vi "Link.vi"(0 "Tosca in":refnum<class "Parameters.lvclass">, 11 "error in (no error)":errorcluster) -> (4 "Tosca out":refnum<class "Parameters.lvclass">, 15 "error out":errorcluster)   [LabVIEW 2020, in "Parameters.lvclass"]
uses:
  Parameters.lvclass
  Parameters.lvclass/Parameters.ctl
  State/State.lvclass
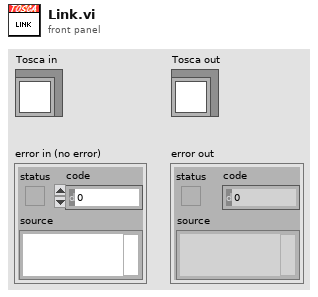
[diagram p1: front panel]
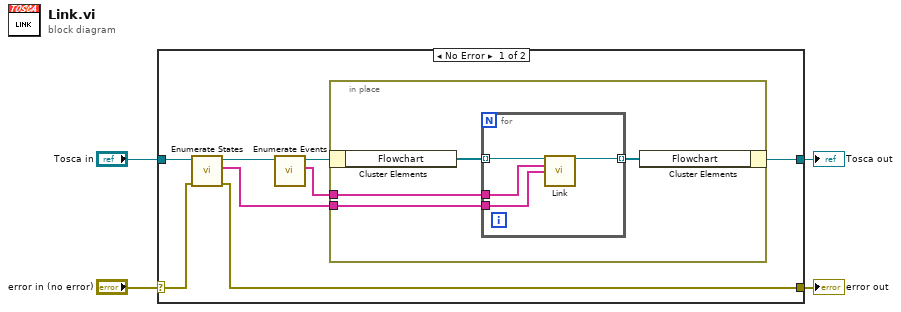
[diagram p0: block diagram]
diagram:
  n1 = case shown="No Error" "error in (no error)" {
    selector: "error in (no error)" -> [w11 w22]
    tunnel: [w10 w22] -> w3
    tunnel: [w8 w21] -> w1
    tunnel: "Tosca in" -> [w12 w21]
    frame No Error {
      n2 = call "Enumerate States.vi"("error in (no error)"=w11, "Tosca in"=w12) -> ("error out"=w10:errorcluster, "Names"=w9:string[], "Tosca out"=w7:refnum<class "Parameters.lvclass">)  [unwired: 7 in]
      n3 = call "Enumerate Events.vi"("Tosca in"=w7) -> ("Event names"=w5:string[], "Tosca out"=w6:refnum<class "Parameters.lvclass">)  [unwired: 8 in, 1 out]
      n4 = in-place {
        in-place-border: w9 -> [w14]
        in-place-border: w5 -> [w13]
        n5 = in-place-cluster #1(w6) -> ("Flowchart"=w16:refnum<class "State.lvclass">[])
        n6 = for {
          tunnel: w16 -> [w20] mode=indexing
          tunnel: [w19] -> w15 mode=indexing
          tunnel: w14 -> [w18]
          tunnel: w13 -> [w17]
          n7 = call "Link.vi"("State in"=w20, "Event Names"=w17, "State Names"=w18) -> ("State out"=w19:refnum<class "State.lvclass">)  [unwired: 11 in, 1 out]
        }
        n8 = in-place-cluster #1("Flowchart"=w15) -> (w8:refnum<class "Parameters.lvclass">)
      }
    }
    frame Error {
    }
  }
  "error out" <- w3
  "Tosca out" <- w1
